vi "Obtain Request Events.vi"(8 "error in (no error)":errorcluster, 10 "Create New? (F)":bool) -> (0 "error out":errorcluster, 2 "Panther Dashboard Request Events":T1)   [LabVIEW 2020, in "Panther Dashboard.lvlib"]
doc: "This VI Obtains/Creates the Requests events that will be used for other modules to communicate with the module that owns this VI. These Requests events will be accessed only via Public API methods for this module.\n\n<b>NOTE</b>: The contents of this VI are automatically generated and modified by the <b>Tools > Delacor > DQMH</b> utilities. Consider using those utilities instead of making your own modifications to this VI.\n_____\nBased on DQMH Project Template 6.1.0.94."
uses:
  Panther Dashboard.lvlib
  Request Events--cluster.ctl
  Stop Argument--cluster.ctl
  Show Panel Argument--cluster.ctl
  Hide Panel Argument--cluster.ctl
  Get Module Execution Status Argument--cluster.ctl
  Show Diagram Argument--cluster.ctl
  Scan DQMH Modules Argument--cluster.ctl
  Tree DQMH Selection Argument--cluster.ctl
  Open Module API Tester Argument--cluster.ctl
  Execute Default Event Request Argument--cluster.ctl
  Launch DQMH Scripting Tools Argument--cluster.ctl
  DQMH Tools Menu--enum.ctl
  Generate Project Documentation Argument--cluster.ctl
  Show About Argument--cluster.ctl
  Update Module ID Argument--cluster.ctl
  Save Library Description Argument--cluster.ctl
  Save VI Description Argument--cluster.ctl
  Open Documentation Argument--cluster.ctl
  Save Project Documentation Argument--cluster.ctl
  Register controls Mouse Enter Argument--cluster.ctl
  Load Project From Path Argument--cluster.ctl
  Add DQMH Module to Current Scan Argument--cluster.ctl
  Highlight Item Argument--cluster.ctl
  Update Status Argument--cluster.ctl
  Add new Module by Path Argument--cluster.ctl
  Refresh Module By Name Argument--cluster.ctl
  Remove Module By Name Argument--cluster.ctl
panel:
  # "NOTE: The contents of this VI are automatically generated and modified by the Tools > Delacor > DQMH utilities. Consider using those utilities instead of making your own modifications to this VI."
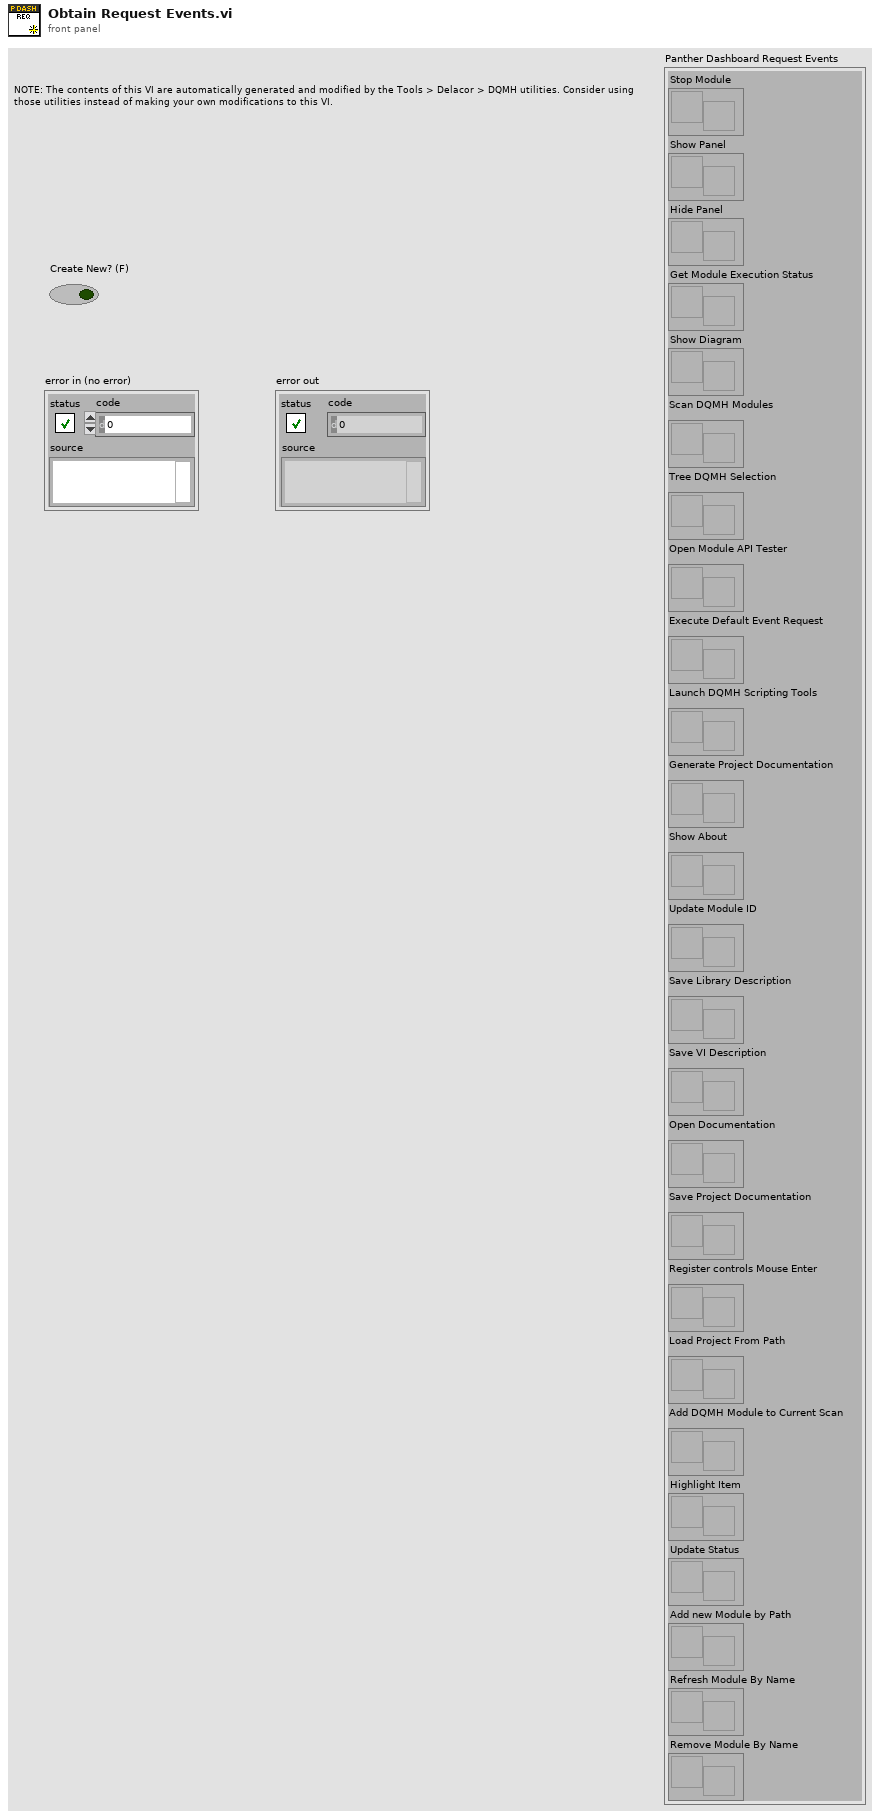
[diagram p1: front panel]
types:
  T1 = typedef "Panther Dashboard.lvlib/Request Events--cluster.ctl" = cluster{"Stop Module":refnum<user-event>, "Show Panel":refnum<user-event>, "Hide Panel":refnum<user-event>, "Get Module Execution Status":refnum<user-event>, "Show Diagram":refnum<user-event>, "Scan DQMH Modules":refnum<user-event>, "Tree DQMH Selection":refnum<user-event>, "Open Module API Tester":refnum<user-event>, "Execute Default Event Request":refnum<user-event>, "Launch DQMH Scripting Tools":refnum<user-event>, "Generate Project Documentation":refnum<user-event>, "Show About":refnum<user-event>, "Update Module ID":refnum<user-event>, "Save Library Description":refnum<user-event>, "Save VI Description":refnum<user-event>, "Open Documentation":refnum<user-event>, "Save Project Documentation":refnum<user-event>, "Register controls Mouse Enter":refnum<user-event>, "Load Project From Path":refnum<user-event>, "Add DQMH Module to Current Scan":refnum<user-event>, "Highlight Item":refnum<user-event>, "Update Status":refnum<user-event>, "Add new Module by Path":refnum<user-event>, "Refresh Module By Name":refnum<user-event>, "Remove Module By Name":refnum<user-event>}
  T2 = typedef "Panther Dashboard.lvlib/Remove Module By Name Argument--cluster.ctl" = cluster{"Module Name":string}
  T3 = typedef "Panther Dashboard.lvlib/Refresh Module By Name Argument--cluster.ctl" = cluster{"Module Name":string}
  T4 = typedef "Panther Dashboard.lvlib/Add new Module by Path Argument--cluster.ctl" = cluster{"Module Folder":path, "Module Name":string}
  T5 = typedef "Panther Dashboard.lvlib/Update Status Argument--cluster.ctl" = cluster{"Status":string}
  T6 = typedef "Panther Dashboard.lvlib/Highlight Item Argument--cluster.ctl" = cluster{"Item Tag":string}
  T7 = typedef "Panther Dashboard.lvlib/Add DQMH Module to Current Scan Argument--cluster.ctl" = cluster{"Include Dependencies":bool}
  T8 = typedef "Panther Dashboard.lvlib/Load Project From Path Argument--cluster.ctl" = cluster{"Project Path":path}
  T9 = typedef "Panther Dashboard.lvlib/Register controls Mouse Enter Argument--cluster.ctl" = cluster{"Boolean":bool}
  T10 = typedef "Panther Dashboard.lvlib/Save Project Documentation Argument--cluster.ctl" = cluster{"Project Description":string}
  T11 = typedef "Panther Dashboard.lvlib/Open Documentation Argument--cluster.ctl" = cluster{"Boolean":bool}
  T12 = typedef "Panther Dashboard.lvlib/Save VI Description Argument--cluster.ctl" = cluster{"VI Description":string}
  T13 = typedef "Panther Dashboard.lvlib/Save Library Description Argument--cluster.ctl" = cluster{"Library Description":string}
  T14 = typedef "Panther Dashboard.lvlib/Update Module ID Argument--cluster.ctl" = cluster{"New ID":i32}
  T15 = typedef "Panther Dashboard.lvlib/Show About Argument--cluster.ctl" = cluster{"Boolean":bool}
  T16 = typedef "Panther Dashboard.lvlib/Generate Project Documentation Argument--cluster.ctl" = cluster{"Boolean":bool}
  T17 = typedef "Panther Dashboard.lvlib/Launch DQMH Scripting Tools Argument--cluster.ctl" = cluster{"Scripting Tool":T18}
  T18 = typedef "Panther Dashboard.lvlib/DQMH Tools Menu--enum.ctl" = enum16{"Create New DQMH Event", "Remove DQMH Event", "Convert DQMH Event", "Rename DQMH Event", "Add New DQMH Module", "Create RT Tester", "Rename DQMH Module", "Validate DQMH Module", "Create DQMH Module Template", "New DQMH  Unit Test", "Add Helper Loop to DQMH Module", "Duplicate Event", "HSE-ify DQMH Module", "Duplicate Module"}
  T19 = typedef "Panther Dashboard.lvlib/Execute Default Event Request Argument--cluster.ctl" = cluster{"Event Name":string}
  T20 = typedef "Panther Dashboard.lvlib/Open Module API Tester Argument--cluster.ctl" = cluster{"Boolean":bool}
  T21 = typedef "Panther Dashboard.lvlib/Tree DQMH Selection Argument--cluster.ctl" = cluster{"Tree Sel":string}
  T22 = typedef "Panther Dashboard.lvlib/Scan DQMH Modules Argument--cluster.ctl" = cluster{"Include Dependencies":bool, "Scan All":bool, "Project":string, "Target":string}
  T23 = typedef "Panther Dashboard.lvlib/Hide Panel Argument--cluster.ctl" = cluster{"Hide Panel?":bool}
  T24 = typedef "Panther Dashboard.lvlib/Show Panel Argument--cluster.ctl" = cluster{"Show Panel?":bool}
  T25 = typedef "Panther Dashboard.lvlib/Show Diagram Argument--cluster.ctl" = cluster{"Debug?":bool}
  T26 = typedef "Panther Dashboard.lvlib/Get Module Execution Status Argument--cluster.ctl" = cluster{"Running?":bool}
  T27 = typedef "Panther Dashboard.lvlib/Stop Argument--cluster.ctl" = cluster{"Origin":string, "Exit via Stop Module Req?":bool, "Wait for Module to stop?":bool}
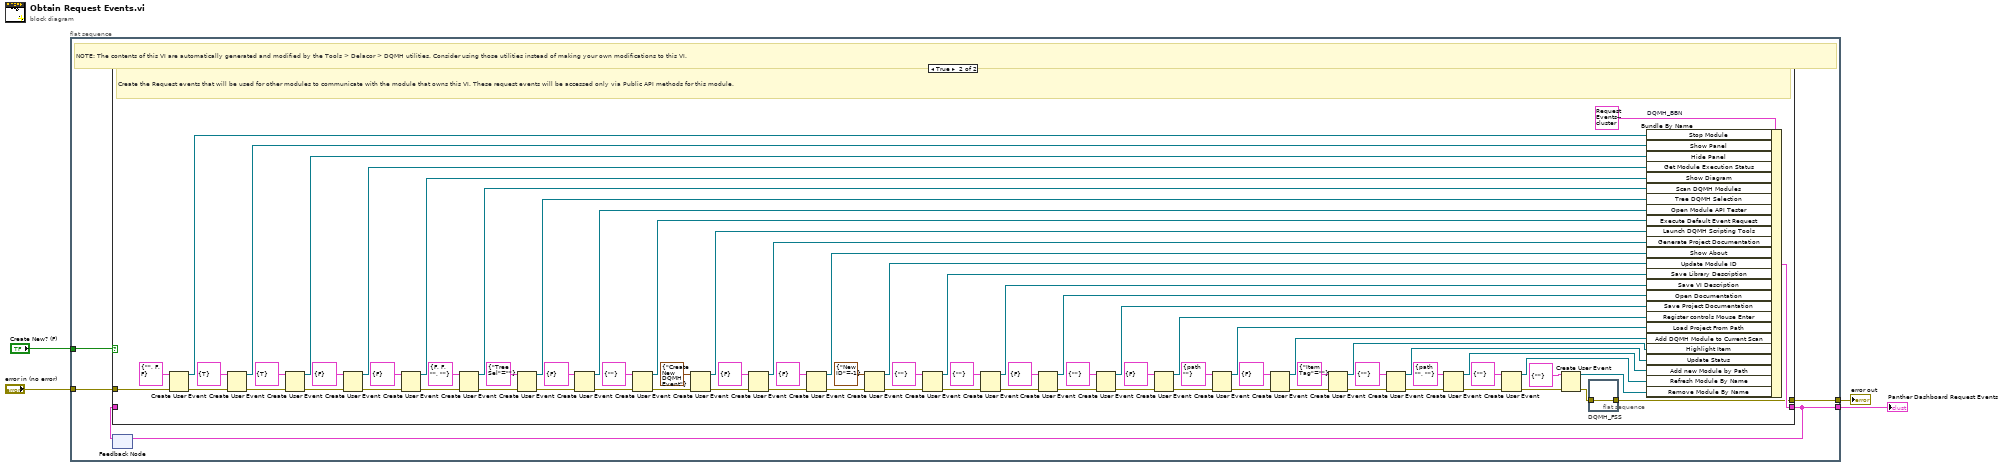
[diagram p0: block diagram]
diagram:
  n1 = flat-sequence {
    tunnel: [w9] -> w4
    tunnel: "error in (no error)" -> [w8]
    tunnel: [w6] -> w2
    tunnel: "Create New? (F)" -> [w5]
    frame #0 {
      # "NOTE: The contents of this VI are automatically generated and modified by the Tools > Delacor > DQMH utilities. Consider using those utilities instead of making your own modifications to this VI."
      n2 = feedback #1() -> (w7:T1)  [unwired: 1 in]
      n3 = case shown="True" w5 {
        tunnel: [w10 w80] -> w9
        tunnel: w8 -> [w10 w90]
        tunnel: [w11 w87] -> w6
        tunnel: w7 -> [w11 _]
        frame False {
          # "Obtain the Request events that were created in a previous call to this VI."
        }
        frame True {
          # "Create the Request events that will be used for other modules to communicate with the module that owns this VI. These request events will be accessed only via Public API methods for this module."
          n4 = Create User Event(user event datatype=T27 {"Origin"="", "Exit via Stop Module Req?"=FALSE, "Wait for Module to stop?"=FALSE} ("Stop Argument"), error in=w90) -> (user event=w88:refnum<user-event>, error out=w85:errorcluster)
          n5 = Create User Event(user event datatype=T24 {"Show Panel?"=TRUE} ("Show Panel Argument"), error in=w85) -> (user event=w84:refnum<user-event>, error out=w83:errorcluster)
          n6 = Create User Event(user event datatype=T23 {"Hide Panel?"=TRUE} ("Hide Panel Argument"), error in=w83) -> (user event=w82:refnum<user-event>, error out=w81:errorcluster)
          n7 = Create User Event(user event datatype=T26 {"Running?"=FALSE} ("Get Module Execution Status Argument"), error in=w81) -> (user event=w78:refnum<user-event>, error out=w79:errorcluster)
          n8 = Create User Event(user event datatype=T25 {"Debug?"=FALSE} ("Show Diagram Argument"), error in=w79) -> (user event=w75:refnum<user-event>, error out=w76:errorcluster)
          n9 = Create User Event(user event datatype=T22 {"Include Dependencies"=FALSE, "Scan All"=FALSE, "Project"="", "Target"=""} ("Scan DQMH Modules Argument"), error in=w76) -> (user event=w70:refnum<user-event>, error out=w71:errorcluster)
          n10 = Create User Event(user event datatype=T21 {"Tree Sel"=""} ("Tree DQMH Selection Argument"), error in=w71) -> (user event=w67:refnum<user-event>, error out=w68:errorcluster)
          n11 = Create User Event(user event datatype=T20 {"Boolean"=FALSE} ("Open Module API Tester Argument"), error in=w68) -> (user event=w64:refnum<user-event>, error out=w65:errorcluster)
          n12 = Create User Event(user event datatype=T19 {"Event Name"=""} ("Execute Default Event Request Argument"), error in=w65) -> (user event=w61:refnum<user-event>, error out=w62:errorcluster)
          n13 = Create User Event(user event datatype=T17 {"Scripting Tool"=enum."Create New DQMH Event"} ("Launch DQMH Scripting Tools Argument"), error in=w62) -> (user event=w58:refnum<user-event>, error out=w59:errorcluster)
          n14 = Create User Event(user event datatype=T16 {"Boolean"=FALSE} ("Generate Project Documentation Argument"), error in=w59) -> (user event=w55:refnum<user-event>, error out=w56:errorcluster)
          n15 = Create User Event(user event datatype=T15 {"Boolean"=FALSE} ("Show About Argument"), error in=w56) -> (user event=w52:refnum<user-event>, error out=w53:errorcluster)
          n16 = Create User Event(user event datatype=T14 {"New ID"=-1} ("Update Module ID Argument"), error in=w53) -> (user event=w49:refnum<user-event>, error out=w50:errorcluster)
          n17 = Create User Event(user event datatype=T13 {"Library Description"=""} ("Save Library Description Argument"), error in=w50) -> (user event=w46:refnum<user-event>, error out=w47:errorcluster)
          n18 = Create User Event(user event datatype=T12 {"VI Description"=""} ("Save VI Description Argument"), error in=w47) -> (user event=w43:refnum<user-event>, error out=w44:errorcluster)
          n19 = Create User Event(user event datatype=T11 {"Boolean"=FALSE} ("Open Documentation Argument"), error in=w44) -> (user event=w40:refnum<user-event>, error out=w41:errorcluster)
          n20 = Create User Event(user event datatype=T10 {"Project Description"=""} ("Save Project Documentation Argument"), error in=w41) -> (user event=w37:refnum<user-event>, error out=w38:errorcluster)
          n21 = Create User Event(user event datatype=T9 {"Boolean"=FALSE} ("Register controls Mouse Enter Argument"), error in=w38) -> (user event=w34:refnum<user-event>, error out=w35:errorcluster)
          n22 = Create User Event(user event datatype=T8 {"Project Path"=path ""} ("Load Project From Path Argument"), error in=w35) -> (user event=w31:refnum<user-event>, error out=w32:errorcluster)
          n23 = Create User Event(user event datatype=T7 {"Include Dependencies"=FALSE} ("Add DQMH Module to Current Scan Argument"), error in=w32) -> (user event=w28:refnum<user-event>, error out=w29:errorcluster)
          n24 = Create User Event(user event datatype=T6 {"Item Tag"=""} ("Highlight Item Argument"), error in=w29) -> (user event=w25:refnum<user-event>, error out=w26:errorcluster)
          n25 = Create User Event(user event datatype=T5 {"Status"=""} ("Update Status Argument"), error in=w26) -> (user event=w22:refnum<user-event>, error out=w23:errorcluster)
          n26 = Create User Event(user event datatype=T4 {"Module Folder"=path "", "Module Name"=""} ("Add new Module by Path Argument"), error in=w23) -> (user event=w19:refnum<user-event>, error out=w20:errorcluster)
          n27 = Create User Event(user event datatype=T3 {"Module Name"=""} ("Refresh Module By Name Argument"), error in=w20) -> (user event=w16:refnum<user-event>, error out=w17:errorcluster)
          n28 = Create User Event(user event datatype=T2 {"Module Name"=""} ("Remove Module By Name Argument"), error in=w17) -> (user event=w13:refnum<user-event>, error out=w14:errorcluster)
          n29 = flat-sequence "DQMH_FSS" {
            tunnel: w14 -> [w91]
            tunnel: [w91] -> w80
            frame #0 {
            }
          }
          n30 = Bundle By Name "DQMH_BBN"(cluster=T1 {"Stop Module"=refnum, "Show Panel"=refnum, "Hide Panel"=refnum, "Get Module Execution Status"=refnum, "Show Diagram"=refnum, "Scan DQMH Modules"=refnum, "Tree DQMH Selection"=refnum, "Open Module API Tester"=refnum, "Execute Default Event Request"=refnum, "Launch DQMH Scripting Tools"=refnum, "Generate Project Documentation"=refnum, "Show About"=refnum, "Update Module ID"=refnum, "Save Library Description"=refnum, "Save VI Description"=refnum, "Open Documentation"=refnum, "Save Project Documentation"=refnum, "Register controls Mouse Enter"=refnum, "Load Project From Path"=refnum, "Add DQMH Module to Current Scan"=refnum, "Highlight Item"=refnum, "Update Status"=refnum, "Add new Module by Path"=refnum, "Refresh Module By Name"=refnum, "Remove Module By Name"=refnum} ("output cluster"), "Stop Module"=w88, "Show Panel"=w84, "Hide Panel"=w82, "Get Module Execution Status"=w78, "Show Diagram"=w75, "Scan DQMH Modules"=w70, "Tree DQMH Selection"=w67, "Open Module API Tester"=w64, "Execute Default Event Request"=w61, "Launch DQMH Scripting Tools"=w58, "Generate Project Documentation"=w55, "Show About"=w52, "Update Module ID"=w49, "Save Library Description"=w46, "Save VI Description"=w43, "Open Documentation"=w40, "Save Project Documentation"=w37, "Register controls Mouse Enter"=w34, "Load Project From Path"=w31, "Add DQMH Module to Current Scan"=w28, "Highlight Item"=w25, "Update Status"=w22, "Add new Module by Path"=w19, "Refresh Module By Name"=w16, "Remove Module By Name"=w13) -> (w87:T1)
        }
      }
      n31 = feedback-in #1(w6) -> ()
    }
  }
  "Panther Dashboard Request Events" <- w2
  "error out" <- w4
